vi "Create Table's Headers.vi"(0 "Data":dynamicdata(graph)) -> (1 "Row Headers":string[](array[string]), 2 "Column Headers":string[](array[string]), 3 "Date of data":string, 4 "Display Date":bool)   [LabVIEW 2020, in "NI_ReportGenerationToolkit.lvlib"]
uses:
  <vilib>/addons/_office/NI_ReportGenerationToolkit.lvlib
  Instance           2 30Saved   Create Table's Headers .vi
  Instance           1 30Saved   Create Table's Headers .vi
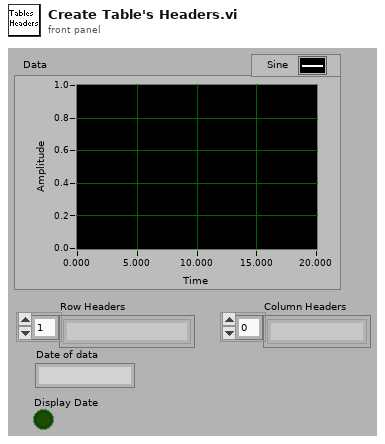
[diagram p1: front panel]
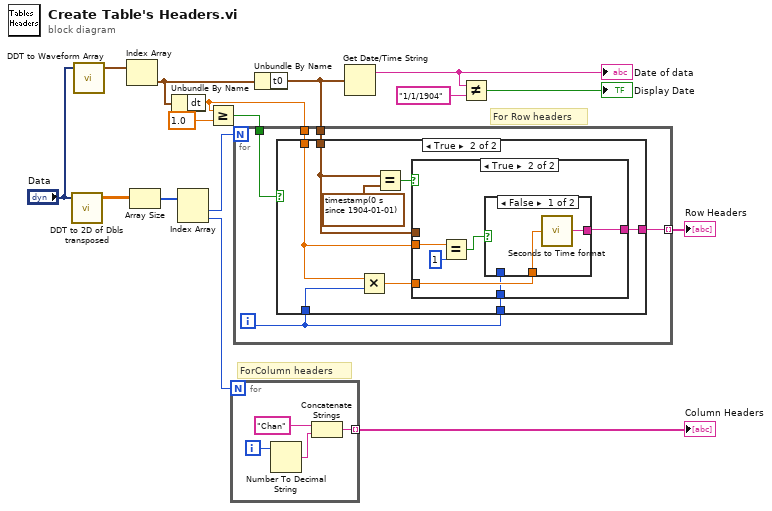
[diagram p0: block diagram]
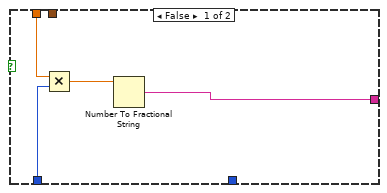
[diagram p2: hidden frame]
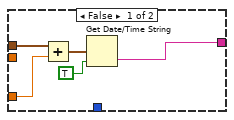
[diagram p3: hidden frame]
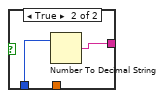
[diagram p4: hidden frame]
diagram:
  # "ForColumn headers"
  # "For Row headers"
  n1 = call "DDT to 2D of Dbls transposed.vi"("Dynamic Data Type"="Data") -> ("2D"=w15:dbl[][])  [unwired: 3 in]
  n2 = call "DDT to Waveform Array.vi"("Dynamic Data Type"="Data") -> ("Array of Waveforms"=w11:waveform(dbl)[])  [unwired: 3 in]
  n3 = Index Array(array=w11) -> (element=w7:waveform(dbl))  [unwired: 1 in]
  n4 = Array Size(array=w15) -> (size(s)=w14:i32[])
  n5 = Unbundle By Name(w7) -> ("dt"=w6:dbl)
  n6 = Index Array(array=w14) -> (element #1=w13:i32, element #2=w1:i32)  [unwired: 2 in]
  n7 = Greater Or Equal?(x=w6, y=1.0) -> (x >= y?=w8:bool)
  n8 = for {
    N: w1 -> [_]
    tunnel: [w17] -> w16 mode=indexing
    i -> [w19]
    n9 = Number To Decimal String(number=w19) -> (decimal integer string=w18:string)  [unwired: 1 in]
    n10 = Concatenate Strings("Chan", w18) -> (w17:string)
  }
  "Column Headers" <- w16
  n11 = Unbundle By Name(w7) -> ("t0"=w5:timestamp)
  n12 = for {
    N: w13 -> [_]
    tunnel: [w25] -> w10 mode=indexing
    tunnel: w8 -> [w24]
    tunnel: w5 -> [w23]
    tunnel: w6 -> [w22]
    i -> [w21]
    n13 = case shown="True" w24 {
      tunnel: w21 -> [w28 w37]
      tunnel: [w26 w33] -> w25
      tunnel: w23 -> [_ w32]
      tunnel: w22 -> [w29 w31]
      tunnel: w21 -> [_ w30]
      frame False {
        n14 = Multiply(x=w29, y=w28) -> (x*y=w27:dbl)
        n15 = Number To Fractional String(number=w27) -> (F-format string=w26:string)  [unwired: 3 in]
      }
      frame True {
        n16 = Multiply(x=w31, y=w37) -> (x*y=w34:dbl)
        n17 = Equal?(x=w32, y=timestamp(0 s since 1904-01-01)) -> (x = y?=w35:bool)
        n18 = case shown="True" w35 {
          tunnel: w34 -> [w42 w48]
          tunnel: [w38 w47] -> w33
          tunnel: w32 -> [w39 _]
          tunnel: w31 -> [_ w46]
          tunnel: w30 -> [_ w43]
          frame False {
            n19 = Add(x=w39, y=w42) -> (x+y=w40:timestamp)
            n20 = Get Date/Time String(seconds (now)=w40, want seconds? (F)=TRUE) -> (time string=w38:string)  [unwired: 1 in, 1 out]
          }
          frame True {
            n21 = Equal?(x=w46, y=1) -> (x = y?=w44:bool)
            n22 = case shown="False" w44 {
              tunnel: w48 -> [w50 _]
              tunnel: [w49 w51] -> w47
              tunnel: w43 -> [_ w52]
              frame False {
                n23 = call <vilib>:"Seconds to Time format.vi"("No of seconds"=w50) -> ("Time output"=w49:string)
              }
              frame True {
                n24 = Number To Decimal String(number=w52) -> (decimal integer string=w51:string)  [unwired: 1 in]
              }
            }
          }
        }
      }
    }
  }
  "Row Headers" <- w10
  n25 = Get Date/Time String(seconds (now)=w5) -> (date string=w4:string)  [unwired: 2 in, 1 out]
  "Date of data" <- w4
  n26 = Not Equal?(x=w4, y="1/1/1904") -> (x != y?=→"Display Date":bool)
